vi "8164B Chassis Self-test.vi"(8 "error in":errorcluster, 10 "slots":string[](array[string]), 11 "KeySight 8164B control in":T1) -> (0 "error out":errorcluster, 2 "error code":u32, 3 "KeySight 8164B control out":T1)   [LabVIEW 2018, in "KeySight 8164B LAN InstrLib.lvlib"]
uses:
  KeySight 8164B LAN InstrLib.lvlib
  typedefs/KeySight 8164B control.ctl
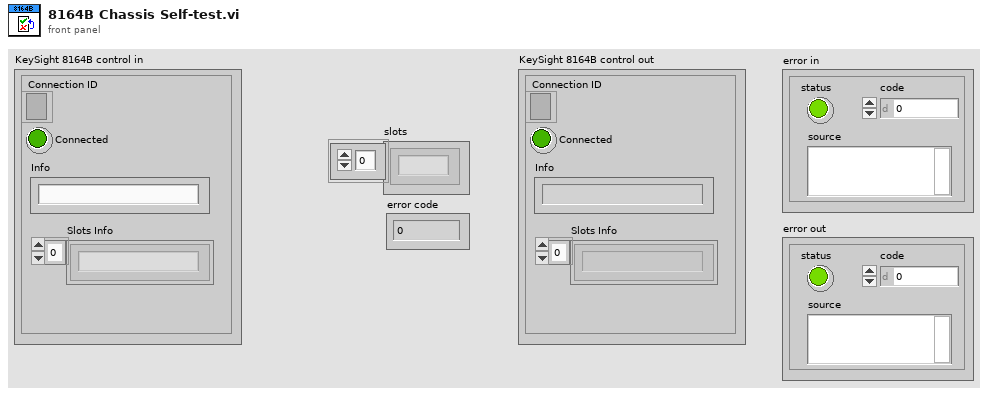
[diagram p1: front panel]
types:
  T1 = typedef "KeySight 8164B LAN InstrLib.lvlib/KeySight 8164B control.ctl" = cluster{"Connection ID":refnum<k5>, "Connected":bool, "Info":string, "Slots Info":string[]}
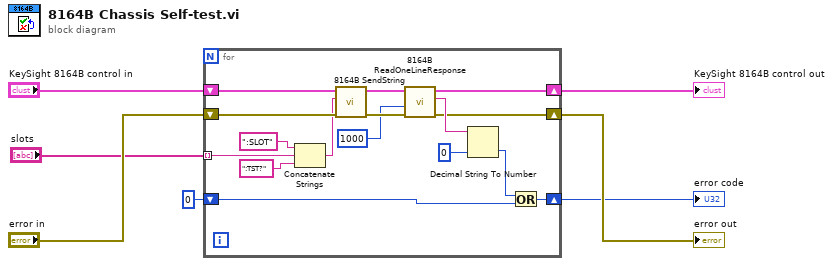
[diagram p0: block diagram]
diagram:
  n1 = for {
    shift-right: [w16] -> w5
    shift-left: "KeySight 8164B control in" -> [w23]
    shift-right: [w15] -> w4
    shift-left: "error in" -> [w22]
    shift-right: [w12] -> w2
    shift-left: u32 0 -> [w13]
    tunnel: "slots" -> [w8] mode=indexing
    n2 = Concatenate Strings(":SLOT", w8, ":TST?") -> (w9:string)
    n3 = call "8164B SendString.vi"("error in"=w22, "CMD"=w9, "KeySight 8164B control in"=w23) -> ("error out"=w20:errorcluster, "KeySight 8164B control out"=w21:T1)  [unwired: 7 in]
    n4 = call "8164B ReadOneLineResponse.vi"("error in"=w20, "timeout ms"=1000 ("timeout ms (25000)"), "KeySight 8164B control in"=w21) -> ("error out"=w15:errorcluster, "OneLineResponse"=w19:string, "KeySight 8164B control out"=w16:T1)  [unwired: 6 in]
    n5 = Decimal String To Number(string=w19, default (0L)=u32 0 ("default (0 I32)")) -> (number=w14:u32)  [unwired: 1 in, 1 out]
    n6 = Or(x=w14, y=w13) -> (x .or. y?=w12:u32)
  }
  "KeySight 8164B control out" <- w5
  "error out" <- w4
  "error code" <- w2
